vi "ZLUTStepRange.vi"() -> ()   [LabVIEW 2011]
uses:
  Main/GlobalVariables.vi
panel:
  in  "Tracking Config.ZLUT Bias correction planes":i32
  in  "Steps":i32[](array[numeric])=[100, 50, 30, 20, 15, 10]
  in  "Distance":dbl=3.0
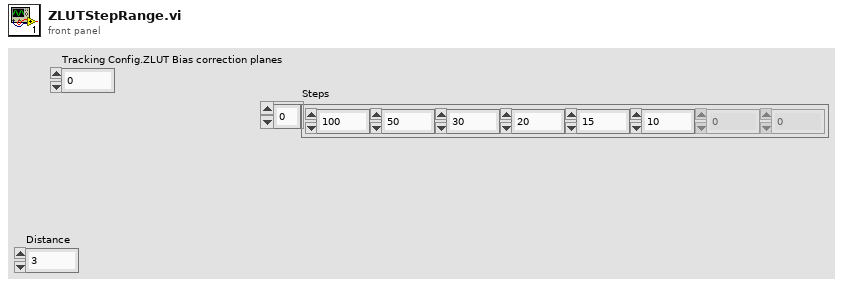
[diagram p1: front panel]
types:
  T1 = enum16{"big-endian, network order", "native, host order", "little-endian"}
  T2 = typedef "MeasureConfigType.ctl" = cluster{"Bead locations":cluster{"X":i32, "Y":i32}[], "ROI":i32, "Experiment base path":path, "Image output subdir":string, "Output mode":T3, "Traces output subdir":string, "QTrk Settings":T4, "Tracking Config":T5, "Experiment Name":string, "Program":T8, "ZLUT":sgl[][][], "Camera settings":T15, "Experiment Script":string, "Max frames in memory":i32, "Save traces as binary":bool, "Pixel Calibration Gain Image":string, "Pixel Calibration Offset Image":string, "Use pixel calibration images":bool, "Internal camera settings":string, "Trace write interval":i32}
  T3 = typedef "MeasureConfigOutputMode.ctl" = enum16{"None", "Track", "SaveImages"}
  T4 = typedef "QTrkSettings.ctl" = cluster{"Image width":i32, "Image height":i32, "Number of threads (CPU based)":i32, "CUDA Device":i32, "COM Background correction factor":sgl, "ZLUT MinRadius":sgl, "ZLUT Radial sample density":sgl, "ZLUT Angular sample density":sgl, "ZLUT ROI Coverage":sgl, "QI Iterations":i32, "QI MinRadius":sgl, "QI Radial sample density":sgl, "QI Angular sample density":sgl, "QI ROI Coverage":sgl, "QI Angular Step \nIteration Factor":sgl, "XCOR Profile Length":i32, "XCOR Profile Width":i32, "XCOR Iterations":i32, "Gaussian 2D Fit Iterations":i32, "Gaussian 2D Sigma (pixels)":sgl, "Downsample":i32}
  T5 = typedef "TrackingConfigType.ctl" = cluster{"Number of steps":i32, "ZLUT stepsize (um)":sgl, "Z correction factor":sgl, "Start piezo Z (um)":sgl, "Pixel size (nm)":sgl, "2D Localization Type":T6, "Z Command (None)":T7, "Z Piezo scale":bool, "ZLUT Building\nimages per frame":i32, "ZLUT Bias correction planes":i32}
  T6 = typedef "QTrkLocalizationType.ctl" = enum16{"Center-of-Mass", "1D Cross-Correlation", "Quadrant Interpolation", "Gaussian 2D MLE", "QI + ZLUTAlign", "ZLUTAlign", "QI + FourierLUT"}
  T7 = typedef "QTrkZCommandType.ctl" = enum16{"Nothing", "ComputeZ"}
  T8 = typedef "ExperimentProgramType.ctl" = cluster{"Commands":T9[], "Motor Axis accuracy conditions":T12, "Axis flags":T14}
  T9 = typedef "ExProgCommandType.ctl" = cluster{"cmd":T10, "axis":T11, "value/pos":dbl, "speed":dbl, "name":string}
  T10 = typedef "ExProgCommandEnumType.ctl" = enum16{"wait", "move", "acquire", "idle", "rmove", "when", "section", "stop"}
  T11 = typedef "MotorAxisEnum.ctl" = enum16{"no axis", "magrot", "magpos", "px", "py", "pz", "camx", "camy"}
  T12 = typedef "MotorPosType.ctl" = cluster{"Magnet Z":dbl, "Magnet rotation":dbl, "Camera":T13, "Piezo XY":T13, "Piezo Z":dbl, "Coil XY":T13}
  T13 = typedef "XYf.ctl" = cluster{"X":sgl, "Y":sgl}
  T14 = typedef "MotorPosFlagsType.ctl" = cluster{"Magnet Z":bool, "Magnet rotation":bool, "Camera":cluster{"X":bool, "Y":bool}, "Piezo XY":cluster{"X":bool, "Y":bool}, "Piezo Z":bool, "Coil XY":cluster{"X":bool, "Y":bool}}
  T15 = typedef "GenericCameraConfigType.ctl" = cluster{"Framerate (Hz)":i32, "Exposure time (us)":i32, "Image size":cluster{"Width":i32, "Height":i32}, "Number of buffers":i32}
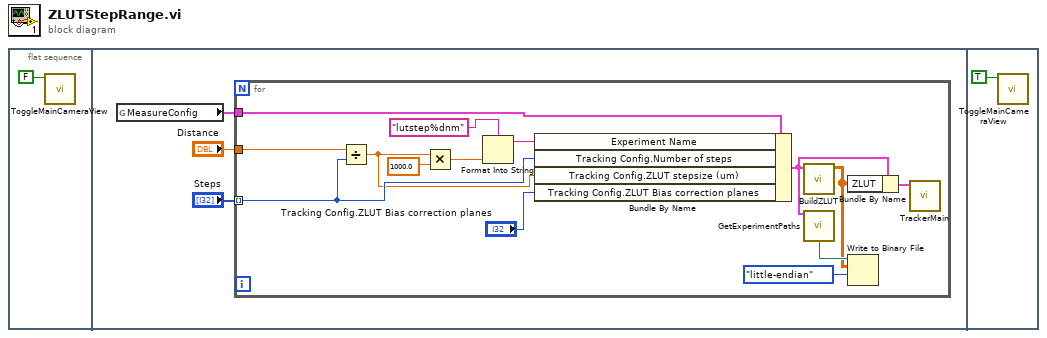
[diagram p0: block diagram]
diagram:
  n1 = flat-sequence {
    frame #0 {
      n2 = call "ToggleMainCameraView.vi"("Enable? (T)"=FALSE) -> ()  [unwired: 11 in]
    }
    frame #1 {
      n3 = global read "GlobalVariables.vi" "MeasureConfig"() -> (w4:T2)
      n4 = for {
        tunnel: w4 -> [w18]
        tunnel: "Steps" -> [w15] mode=indexing
        tunnel: "Distance" -> [w16]
        n5 = Divide(x=w16, y=w15) -> (x/y=w12:dbl)
        n6 = Multiply(x=w12, y=1000.0) -> (x*y=w11:dbl)
        n7 = Format Into String(format string="lutstep%dnm", w11) -> (resulting string=w10:string)  [unwired: 2 in, 1 out]
        n8 = Bundle By Name(cluster=w18, "Experiment Name"=w10, "Tracking Config.Number of steps"=w15, "Tracking Config.ZLUT stepsize (um)"=w12, "Tracking Config.ZLUT Bias correction planes"="Tracking Config.ZLUT Bias correction planes") -> (w9:T2)
        n9 = call "BuildZLUT.vi"("MeasureConfig"=w9) -> ("ZLUT"=w7:sgl[][][])  [unwired: 9 in, 1 out]
        n10 = call "GetExperimentPaths.vi"("MeasureConfig"=w9) -> ("[base]\\[expname].radialzlut"=w8:path)  [unwired: 6 in, 8 out]
        n11 = Bundle By Name(cluster=w9, "ZLUT"=w7) -> (w17:T2)
        n12 = Write to Binary File(file (use dialog)=w8, data=w7, 9:T1."little-endian" ("byte order (0:big-endian, network order)")) -> ()  [unwired: 3 in, 3 out]
        n13 = call "TrackerMain.vi"("MeasureConfig"=w17) -> ()  [unwired: 10 in, 1 out]
      }
    }
    frame #2 {
      n14 = call "ToggleMainCameraView.vi"("Enable? (T)"=TRUE) -> ()  [unwired: 11 in]
    }
  }
